vi "Teleop.vi"(10 "Match Info":T1={"Autonomous Elapsed Seconds"=0.0, "TeleOp Elapsed Seconds"=0.0, "Disabled Elapsed Seconds"=0.0, "Visited Autonomous"=FALSE, "Visited TeleOp"=FALSE, "Visited Disabled"=FALSE, "Autonomous Settings"={"Autonomous Style"=enum."Independent", "VI Refnum"=refnum}}, 11 "Call Context":T2) -> ()   [LabVIEW 2017]
doc: "This VI is called for each TeleOp packet received from the DS where the robot is not disabled. It is often used to read from the joysticks and update I/O or to update setpoints for timed control loops. It should complete and return within 20 milliseconds or it may miss DS packets."
uses:
  <vilib>/Rock Robotics/WPI/DriverStation/WPI_DriverStationDerivedRobotMode.ctl
  <vilib>/Rock Robotics/WPI/DriverStation/WPI_DriverStationMatch Info.ctl
  <vilib>/Rock Robotics/WPI/Utilities/WPI_GetSetVariantRefNum.vi
  981LabViewComponents/Global Arm Variables.vi
  981LabViewComponents/Global Teleop Variables.vi
panel:
  in  "Joystick 1 Trigger Button":bool
  out "Buttons":bool[](array[boolean])
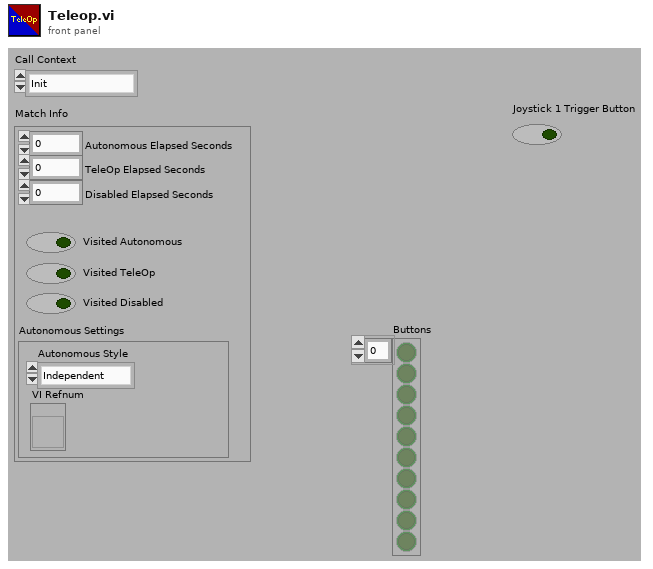
[diagram p1: front panel]
types:
  T1 = typedef "WPI_DriverStationMatch Info.ctl" = cluster{"Autonomous Elapsed Seconds":dbl, "TeleOp Elapsed Seconds":dbl, "Disabled Elapsed Seconds":dbl, "Visited Autonomous":bool, "Visited TeleOp":bool, "Visited Disabled":bool, "Autonomous Settings":cluster{"Autonomous Style":enum16{"Iterative", "Independent"}, "VI Refnum":refnum<vi>}}
  T2 = typedef "WPI_DriverStationDerivedRobotMode.ctl" = enum16{"Init", "Execute", "Stop"}
  T3 = typedef "WPI_JoystickDevRef.ctl" = cluster{"Device":T4}
  T4 = typedef "WPI_JoystickDeviceEnum.ctl" = enum16{"USB 0", "USB 1", "USB 2", "USB 3", "USB 4", "USB 5"}
  T5 = typedef "WPI_RobotDriveDevRef.ctl" = cluster{"DevStatus":errorcluster, "Motors[]":T6[], "Square Inputs":bool, "Max Output":dbl}
  T6 = typedef "WPI_MotorControlDeviceRef.ctl" = cluster{"DeviceStatus":errorcluster, "Type":T7, "PWM":cluster{"PWM Channel":T8, "DeadBand":T9}, "CAN":cluster{"Device Number":u8, "SetOutput VI Ref":variant, "GetOutput VI Ref":variant, "Enable VI Ref":variant, "Disable VI Ref":variant, "Data":variant}, "Invert":bool, "DIO PWM":cluster{"PWM \"Enable\" Channel":T8, "DIOChannel":T10, "PWM Rate":dbl}}
  T7 = typedef "WPI_MotorControlType.ctl" = enum16{"PWM", "CAN", "DIO PWM"}
  T8 = typedef "FPGA_DIOPWMChannel.ctl" = enum8{"PWM 0", "PWM 1", "PWM 2", "PWM 3", "PWM 4", "PWM 5", "PWM 6", "PWM 7", "PWM 8", "PWM 9", "PWM MXP 0", "PWM MXP 1", "PWM MXP 2", "PWM MXP 3", "PWM MXP 4", "PWM MXP 5", "PWM MXP 6", "PWM MXP 7", "PWM MXP 8", "PWM MXP 9", "Invalid"}
  T9 = typedef "WPI_PWMDeadband.ctl" = cluster{"Name":string, "maxPositivePwm":i32, "minPositivePwm":i32, "centerPwm":i32, "maxNegativePwm":i32, "minNegativePwm":i32, "angularRange":u16}
  T10 = typedef "FPGA_DIOChannel.ctl" = enum8{"DIO 0", "DIO 1", "DIO 2", "DIO 3", "DIO 4", "DIO 5", "DIO 6", "DIO 7", "DIO 8", "DIO 9", "DIO MXP 0", "DIO MXP 1", "DIO MXP 2", "DIO MXP 3", "DIO MXP 4", "DIO MXP 5", "DIO MXP 6", "DIO MXP 7", "DIO MXP 8", "DIO MXP 9", "DIO MXP 10", "DIO MXP 11", "DIO MXP 12", "DIO MXP 13", "DIO MXP 14", "DIO MXP 15", "SPI Port CS1", "SPI Port CS2", "SPI Port CS3", "SPI Port MISO", "SPI Port MOSI", "Invalid"}
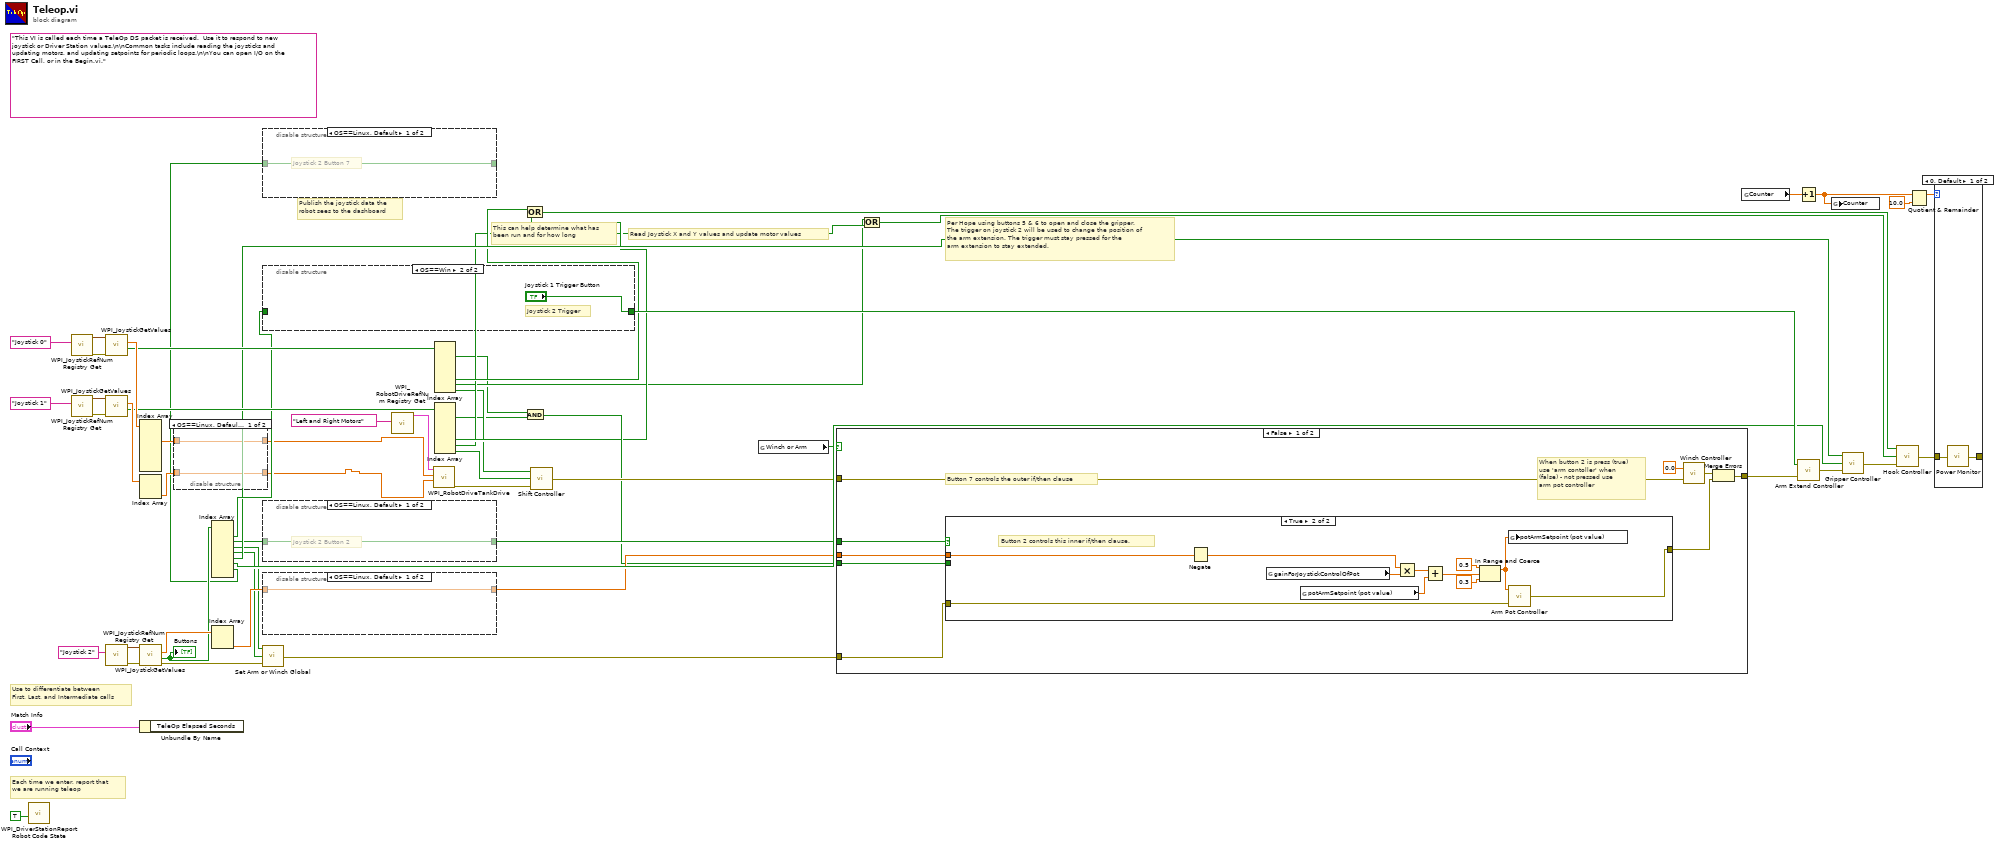
[diagram p0: block diagram]
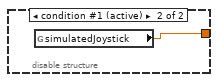
[diagram p2: hidden frame]
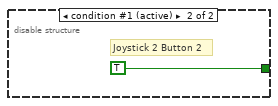
[diagram p3: hidden frame]
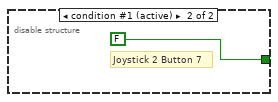
[diagram p4: hidden frame]
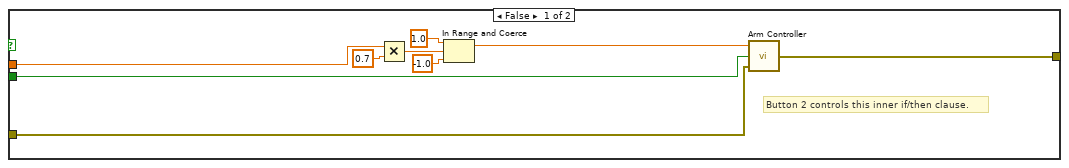
[diagram p5: hidden frame]
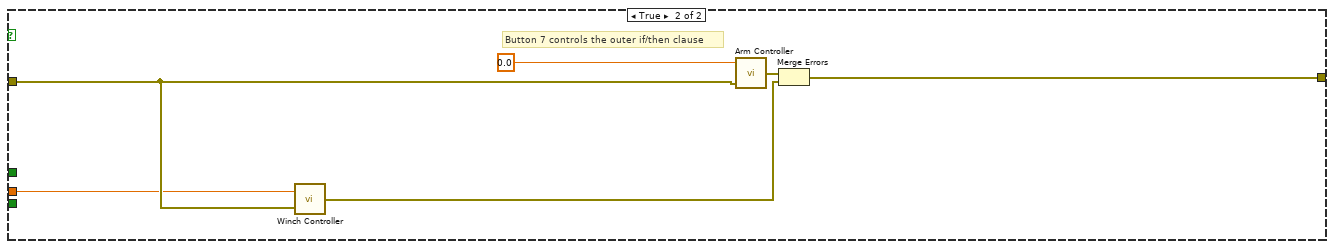
[diagram p6: hidden frame]
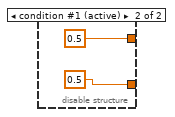
[diagram p9: hidden frame]
diagram:
  (unwired) "This VI is called each time a TeleOp DS packet is received.  Use it to respond to new joystick or Driver Station values.\n\nCommon tasks include reading the joysticks and updating motors, and updating setpoints for periodic loops.\n\nYou can open I/O on the FIRST Call, or in the Begin.vi."
  # "Per Hope using buttons 5 & 6 to open and close the gripper.\nThe trigger on joystick 2 will be used to change the position of\nthe arm extension. The trigger must stay pressed for the \narm extension to stay extended."
  # "Publish the joystick data the\nrobot sees to the dashboard"
  # "Each time we enter, report that\nwe are running teleop"
  # "Use to differentiate between\nFirst, Last, and Intermediate calls"
  # "This can help determine what has\nbeen run and for how long"
  # "Read Joystick X and Y values and update motor values"
  n1 = call <vilib>:"WPI_DriverStationReport Robot Code State.vi"("TeleOp"=TRUE ("Autonomous")) -> ()  [unwired: 10 in, 1 out]
  n2 = call <vilib>:"WPI_JoystickRefNum Registry Get.vi"("refnum name"="Joystick 0") -> ("error out"=w11:errorcluster, "JoystickDevRef"=w55:T3)  [unwired: 1 in, 8 out]
  n3 = call <vilib>:"WPI_JoystickRefNum Registry Get.vi"("refnum name"="Joystick 1") -> ("error out"=w7:errorcluster, "JoystickDevRef"=w51:T3)  [unwired: 1 in, 8 out]
  n4 = call <vilib>:"WPI_JoystickGetValues.vi"("error in (no error)"=w11, "JoystickDevRef"=w55) -> ("Buttons"=w41:bool[], "Axes"=w53:dbl[])  [unwired: 5 in, 3 out]
  n5 = call <vilib>:"WPI_JoystickGetValues.vi"("error in (no error)"=w7, "JoystickDevRef"=w51) -> ("Buttons"=w40:bool[], "Axes"=w47:dbl[])  [unwired: 5 in, 3 out]
  n6 = call <vilib>:"WPI_JoystickRefNum Registry Get.vi"("refnum name"="Joystick 2") -> ("error out"=w8:errorcluster, "JoystickDevRef"=w45:T3)  [unwired: 1 in, 8 out]
  n7 = Unbundle By Name("Match Info") -> ()  [unwired: 1 out]
  n8 = Index Array(array=w53) -> (element #2=w50:dbl)  [unwired: 7 in, 6 out]
  n9 = Index Array(array=w47) -> (element #2=w49:dbl)  [unwired: 2 in, 1 out]
  n10 = call <vilib>:"WPI_JoystickGetValues.vi"("error in (no error)"=w8, "JoystickDevRef"=w45) -> ("error out"=w9:errorcluster, "Buttons"=w43:bool[], "Axes"=w44:dbl[])  [unwired: 5 in, 2 out]
  "Buttons" <- w43
  n11 = disable-structure shown="OS==Linux, Default" {
    disable-tunnel: [w60 0.5 ("X axis value")] -> w1
    disable-tunnel: w50 -> [w60 _]
    disable-tunnel: w49 -> [w59 _]
    disable-tunnel: [w59 0.5 ("X axis value")] -> w2
    frame condition #0 {
    }
    frame condition #1 (active) {
    }
  }
  n12 = Index Array(array=w43) -> (element #1=w32:bool, element #2=w24:bool, element #3=w14:bool, element #4=w13:bool, element #5=w28:bool, element #6=w27:bool, element #7=w29:bool)  [unwired: 8 in, 1 out]
  n13 = Index Array(array=w44) -> (element #2=w22:dbl)  [unwired: 2 in, 1 out]
  n14 = disable-structure shown="OS==Linux, Default" {
    disable-tunnel: [w63 FALSE] -> _
    disable-tunnel: w29 -> [w63 _]
    frame condition #0 {
      # "Joystick 2 Button 7"
    }
    frame condition #1 (active) {
      # "Joystick 2 Button 7"
    }
  }
  n15 = disable-structure shown="OS==Win" {
    disable-tunnel: w32 -> [w65 _]
    disable-tunnel: [w65 "Joystick 1 Trigger Button"] -> w31
    frame condition #0 {
      # "Joystick 2 Trigger"
    }
    frame condition #1 (active) {
      # "Joystick 2 Trigger"
    }
  }
  n16 = disable-structure shown="OS==Linux, Default" {
    disable-tunnel: [w67 TRUE] -> w25
    disable-tunnel: w24 -> [w67 _]
    frame condition #0 {
      # "Joystick 2 Button 2"
    }
    frame condition #1 (active) {
      # "Joystick 2 Button 2"
    }
  }
  n17 = disable-structure shown="OS==Linux, Default" {
    disable-tunnel: [w69 w70] -> w23
    disable-tunnel: w22 -> [w69 _]
    frame condition #0 {
    }
    frame condition #1 (active) {
      n18 = global read "Global Arm Variables.vi" "simulatedJoystick"() -> (w70:dbl)
    }
  }
  n19 = call "Set Arm or Winch Global.vi"("error in"=w9, "Button B"=w13, "Button A"=w14) -> ("error out"=w10:errorcluster)
  n20 = call <vilib>:"WPI_RobotDriveRefNum Registry Get.vi"("refnum name"="Left and Right Motors") -> ("RobotDriveDevRef"=w48:T5)  [unwired: 1 in, 9 out]
  n21 = call <vilib>:"WPI_RobotDriveTankDrive.vi"("Right axis value"=w2, "Left axis value"=w1, "RobotDriveDevRef"=w48) -> ("error out"=w42:errorcluster)  [unwired: 6 in, 2 out]
  n22 = Index Array(array=w41) -> (element #1=w4:bool, element #5=w19:bool, element #6=w16:bool, element #7=w6:bool)  [unwired: 7 in, 3 out]
  n23 = Index Array(array=w40) -> (element #1=w3:bool, element #5=w20:bool, element #6=w17:bool, element #7=w5:bool)  [unwired: 7 in, 3 out]
  n24 = Or(x=w19, y=w20) -> (x .or. y?=w18:bool)
  n25 = And(x=w4, y=w3) -> (x .and. y?=w21:bool)
  n26 = call "Shift Controller.vi"("error in"=w42, "Right Trigger"=w5, "Left Trigger"=w6) -> ("error out"=w26:errorcluster)
  n27 = global read "Global Arm Variables.vi" "Winch or Arm"() -> (w12:bool)
  n28 = case shown="False" w12 {
    tunnel: w26 -> [w78 w105]
    tunnel: [w76 w102] -> w30
    tunnel: w25 -> [w75 _]
    tunnel: w10 -> [w74 _]
    tunnel: w23 -> [w73 w100]
    tunnel: w21 -> [w71 _]
    frame False {
      # "Button 7 controls the outer if/then clause"
      # "When button 2 is press (true)\nuse 'arm contoller' when\n(false) - not pressed use\narm pot controller"
      n29 = case shown="True" w75 {
        tunnel: w74 -> [w88 w98]
        tunnel: w73 -> [w84 w89]
        tunnel: [w87 w99] -> w72
        tunnel: w71 -> [w80 _]
        frame False {
          # "Button 2 controls this inner if/then clause."
          n30 = Multiply(x=w84, y=0.7) -> (x*y=w82:dbl)
          n31 = In Range and Coerce(upper limit=1.0, x=w82, lower limit=-1.0) -> (coerced(x)=w81:dbl)  [unwired: 1 out]
          n32 = call "Arm Controller.vi"("error in"=w88, "Button7OnBothJostick1and2"=w80, "Input"=w81) -> ("error out"=w87:errorcluster)
        }
        frame True {
          # "Button 2 controls this inner if/then clause."
          n33 = Negate(x=w89) -> (-x=w90:dbl)
          n34 = global read "Global Arm Variables.vi" "gainForJoystickControlOfPot"() -> (w91:dbl)
          n35 = global read "Global Arm Variables.vi" "potArmSetpoint (pot value)"() -> (w97:dbl)
          n36 = Multiply(x=w90, y=w91) -> (x*y=w96:dbl)
          n37 = Add(x=w96, y=w97) -> (x+y=w95:dbl)
          n38 = In Range and Coerce(upper limit=0.5, x=w95, lower limit=0.3) -> (coerced(x)=w92:dbl)  [unwired: 1 out]
          n39 = global write "Global Arm Variables.vi" "potArmSetpoint (pot value)"(w92) -> ()
          n40 = call "Arm Pot Controller.vi"("error in"=w98, "teleopSetup"=w92) -> ("error out"=w99:errorcluster)  [unwired: 1 in]
        }
      }
      n41 = call "Winch Controller.vi"("error in"=w78, "Input"=0.0) -> ("error out"=w77:errorcluster)
      n42 = Merge Errors(w77, w72) -> (w76:errorcluster)
    }
    frame True {
      # "Button 7 controls the outer if/then clause"
      n43 = call "Winch Controller.vi"("error in"=w105, "Input"=w100) -> ("error out"=w103:errorcluster)
      n44 = call "Arm Controller.vi"("error in"=w105, "Input"=0.0) -> ("error out"=w104:errorcluster)  [unwired: 1 in]
      n45 = Merge Errors(w104, w103) -> (w102:errorcluster)
    }
  }
  n46 = Or(x=w16, y=w17) -> (x .or. y?=w15:bool)
  n47 = global read "Global Teleop Variables.vi" "Counter"() -> (w38:dbl)
  n48 = Increment(x=w38) -> (x+1=w37:dbl)
  n49 = call "Arm Extend Controller.vi"("error in"=w30, "Trigger"=w31) -> ("error out"=w33:errorcluster)
  n50 = global write "Global Teleop Variables.vi" "Counter"(w37) -> ()
  n51 = call "Gripper Controller.vi"("error in"=w33, "Button B"=w27, "Button A"=w28) -> ("error out"=w39:errorcluster)
  n52 = call "Hook Controller.vi"("error in"=w39, "Button B"=w15, "Button A"=w18) -> ("error out"=w34:errorcluster)
  n53 = Quotient & Remainder(x=w37, y=10.0) -> (x-y*floor(x/y)=w35:dbl)  [unwired: 1 out]
  n54 = case shown="0, Default" w35 {
    tunnel: w34 -> [w107 w108]
    tunnel: [w106 w108] -> _
    frame 0, Default {
      n55 = call "Power Monitor.vi"("error in"=w107) -> ("error out"=w106:errorcluster)
    }
    frame 1 {
    }
  }
